vi "StarWarsMelody (SubVI).vi"() -> (3 "Array":dbl[][](array[numeric]))   [LabVIEW 2014]
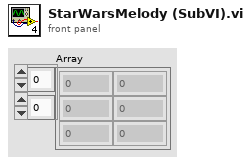
[diagram p1: front panel]
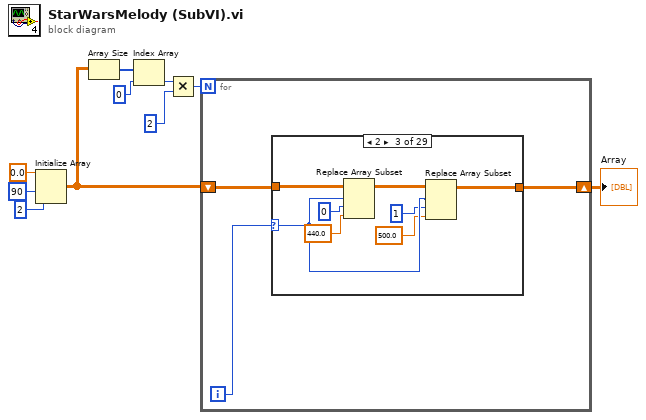
[diagram p0: block diagram]
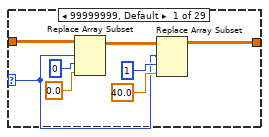
[diagram p2: hidden frame]
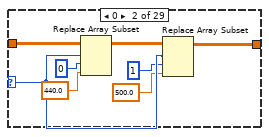
[diagram p3: hidden frame]
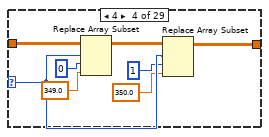
[diagram p4: hidden frame]
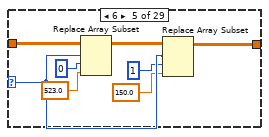
[diagram p5: hidden frame]
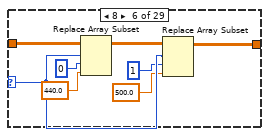
[diagram p6: hidden frame]
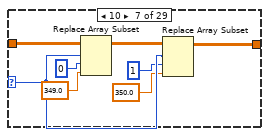
[diagram p7: hidden frame]
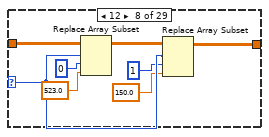
[diagram p8: hidden frame]
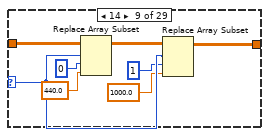
[diagram p9: hidden frame]
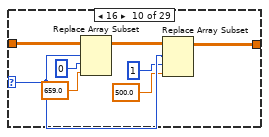
[diagram p10: hidden frame]
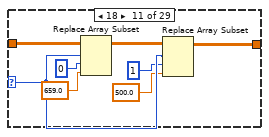
[diagram p11: hidden frame]
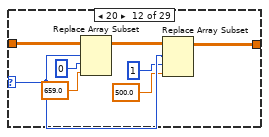
[diagram p12: hidden frame]
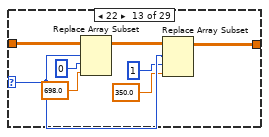
[diagram p13: hidden frame]
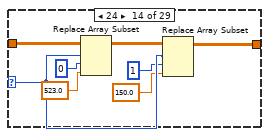
[diagram p14: hidden frame]
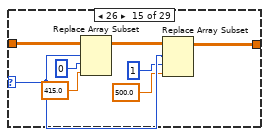
[diagram p15: hidden frame]
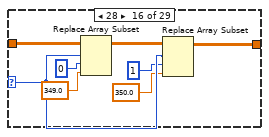
[diagram p16: hidden frame]
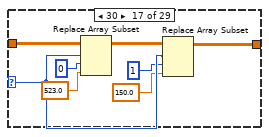
[diagram p17: hidden frame]
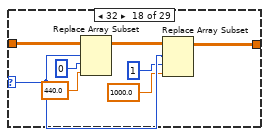
[diagram p18: hidden frame]
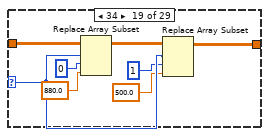
[diagram p19: hidden frame]
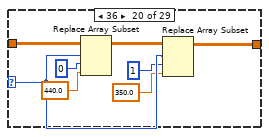
[diagram p20: hidden frame]
diagram:
  n1 = Initialize Array(0.0 ("element"), 90 ("dimension size"), 2 ("dimension size")) -> (w8:dbl[][])
  n2 = Array Size(array=w8) -> (size(s)=w9:i32[])
  n3 = Index Array(array=w9, index=0) -> (element=w3:i32)
  n4 = Multiply(x=w3, y=2) -> (x*y=w4:i32)
  n5 = for {
    N: w4 -> [_]
    shift-right: [w12] -> w1
    shift-left: w8 -> [w13]
    i -> [w11]
    n6 = case shown="2" w11 {
      selector: w11 -> [w14 w25 w33 w41 w49 w57 w65 w73 w81 w89 w97 w105 w113 w121 w129 w137 w145 w153 w161 w169 w177 w185 w193 w201 w209 w217 w225 w233 w241]
      tunnel: w13 -> [w15 w29 w37 w45 w53 w61 w69 w77 w85 w93 w101 w109 w117 w125 w133 w141 w149 w157 w165 w173 w181 w189 w197 w205 w213 w221 w229 w237 w245]
      tunnel: [w16 w22 w30 w38 w46 w54 w62 w70 w78 w86 w94 w102 w110 w118 w126 w134 w142 w150 w158 w166 w174 w182 w190 w198 w206 w214 w222 w230 w238] -> w12
      frame 99999999, Default {
        n7 = Replace Array Subset(array=w15, new element=0.0 ("new element/subarray"), index (row)=w14, index (col)=0 ("disabled index (col)")) -> (w19:dbl[][])
        n8 = Replace Array Subset(array=w19, new element=40.0 ("new element/subarray"), index (row)=w14, index (col)=1 ("disabled index (col)")) -> (w16:dbl[][])
      }
      frame 0 {
        n9 = Replace Array Subset(array=w29, new element=440.0 ("new element/subarray"), index (row)=w25, index (col)=0 ("disabled index (col)")) -> (w26:dbl[][])
        n10 = Replace Array Subset(array=w26, new element=500.0 ("new element/subarray"), index (row)=w25, index (col)=1 ("disabled index (col)")) -> (w22:dbl[][])
      }
      frame 2 {
        n11 = Replace Array Subset(array=w37, new element=440.0 ("new element/subarray"), index (row)=w33, index (col)=0 ("disabled index (col)")) -> (w34:dbl[][])
        n12 = Replace Array Subset(array=w34, new element=500.0 ("new element/subarray"), index (row)=w33, index (col)=1 ("disabled index (col)")) -> (w30:dbl[][])
      }
      frame 4 {
        n13 = Replace Array Subset(array=w45, new element=349.0 ("new element/subarray"), index (row)=w41, index (col)=0 ("disabled index (col)")) -> (w42:dbl[][])
        n14 = Replace Array Subset(array=w42, new element=350.0 ("new element/subarray"), index (row)=w41, index (col)=1 ("disabled index (col)")) -> (w38:dbl[][])
      }
      frame 6 {
        n15 = Replace Array Subset(array=w53, new element=523.0 ("new element/subarray"), index (row)=w49, index (col)=0 ("disabled index (col)")) -> (w50:dbl[][])
        n16 = Replace Array Subset(array=w50, new element=150.0 ("new element/subarray"), index (row)=w49, index (col)=1 ("disabled index (col)")) -> (w46:dbl[][])
      }
      frame 8 {
        n17 = Replace Array Subset(array=w61, new element=440.0 ("new element/subarray"), index (row)=w57, index (col)=0 ("disabled index (col)")) -> (w58:dbl[][])
        n18 = Replace Array Subset(array=w58, new element=500.0 ("new element/subarray"), index (row)=w57, index (col)=1 ("disabled index (col)")) -> (w54:dbl[][])
      }
      frame 10 {
        n19 = Replace Array Subset(array=w69, new element=349.0 ("new element/subarray"), index (row)=w65, index (col)=0 ("disabled index (col)")) -> (w66:dbl[][])
        n20 = Replace Array Subset(array=w66, new element=350.0 ("new element/subarray"), index (row)=w65, index (col)=1 ("disabled index (col)")) -> (w62:dbl[][])
      }
      frame 12 {
        n21 = Replace Array Subset(array=w77, new element=523.0 ("new element/subarray"), index (row)=w73, index (col)=0 ("disabled index (col)")) -> (w74:dbl[][])
        n22 = Replace Array Subset(array=w74, new element=150.0 ("new element/subarray"), index (row)=w73, index (col)=1 ("disabled index (col)")) -> (w70:dbl[][])
      }
      frame 14 {
        n23 = Replace Array Subset(array=w85, new element=440.0 ("new element/subarray"), index (row)=w81, index (col)=0 ("disabled index (col)")) -> (w82:dbl[][])
        n24 = Replace Array Subset(array=w82, new element=1000.0 ("new element/subarray"), index (row)=w81, index (col)=1 ("disabled index (col)")) -> (w78:dbl[][])
      }
      frame 16 {
        n25 = Replace Array Subset(array=w93, new element=659.0 ("new element/subarray"), index (row)=w89, index (col)=0 ("disabled index (col)")) -> (w90:dbl[][])
        n26 = Replace Array Subset(array=w90, new element=500.0 ("new element/subarray"), index (row)=w89, index (col)=1 ("disabled index (col)")) -> (w86:dbl[][])
      }
      frame 18 {
        n27 = Replace Array Subset(array=w101, new element=659.0 ("new element/subarray"), index (row)=w97, index (col)=0 ("disabled index (col)")) -> (w98:dbl[][])
        n28 = Replace Array Subset(array=w98, new element=500.0 ("new element/subarray"), index (row)=w97, index (col)=1 ("disabled index (col)")) -> (w94:dbl[][])
      }
      frame 20 {
        n29 = Replace Array Subset(array=w109, new element=659.0 ("new element/subarray"), index (row)=w105, index (col)=0 ("disabled index (col)")) -> (w106:dbl[][])
        n30 = Replace Array Subset(array=w106, new element=500.0 ("new element/subarray"), index (row)=w105, index (col)=1 ("disabled index (col)")) -> (w102:dbl[][])
      }
      frame 22 {
        n31 = Replace Array Subset(array=w117, new element=698.0 ("new element/subarray"), index (row)=w113, index (col)=0 ("disabled index (col)")) -> (w114:dbl[][])
        n32 = Replace Array Subset(array=w114, new element=350.0 ("new element/subarray"), index (row)=w113, index (col)=1 ("disabled index (col)")) -> (w110:dbl[][])
      }
      frame 24 {
        n33 = Replace Array Subset(array=w125, new element=523.0 ("new element/subarray"), index (row)=w121, index (col)=0 ("disabled index (col)")) -> (w122:dbl[][])
        n34 = Replace Array Subset(array=w122, new element=150.0 ("new element/subarray"), index (row)=w121, index (col)=1 ("disabled index (col)")) -> (w118:dbl[][])
      }
      frame 26 {
        n35 = Replace Array Subset(array=w133, new element=415.0 ("new element/subarray"), index (row)=w129, index (col)=0 ("disabled index (col)")) -> (w130:dbl[][])
        n36 = Replace Array Subset(array=w130, new element=500.0 ("new element/subarray"), index (row)=w129, index (col)=1 ("disabled index (col)")) -> (w126:dbl[][])
      }
      frame 28 {
        n37 = Replace Array Subset(array=w141, new element=349.0 ("new element/subarray"), index (row)=w137, index (col)=0 ("disabled index (col)")) -> (w138:dbl[][])
        n38 = Replace Array Subset(array=w138, new element=350.0 ("new element/subarray"), index (row)=w137, index (col)=1 ("disabled index (col)")) -> (w134:dbl[][])
      }
      frame 30 {
        n39 = Replace Array Subset(array=w149, new element=523.0 ("new element/subarray"), index (row)=w145, index (col)=0 ("disabled index (col)")) -> (w146:dbl[][])
        n40 = Replace Array Subset(array=w146, new element=150.0 ("new element/subarray"), index (row)=w145, index (col)=1 ("disabled index (col)")) -> (w142:dbl[][])
      }
      frame 32 {
        n41 = Replace Array Subset(array=w157, new element=440.0 ("new element/subarray"), index (row)=w153, index (col)=0 ("disabled index (col)")) -> (w154:dbl[][])
        n42 = Replace Array Subset(array=w154, new element=1000.0 ("new element/subarray"), index (row)=w153, index (col)=1 ("disabled index (col)")) -> (w150:dbl[][])
      }
      frame 34 {
        n43 = Replace Array Subset(array=w165, new element=880.0 ("new element/subarray"), index (row)=w161, index (col)=0 ("disabled index (col)")) -> (w162:dbl[][])
        n44 = Replace Array Subset(array=w162, new element=500.0 ("new element/subarray"), index (row)=w161, index (col)=1 ("disabled index (col)")) -> (w158:dbl[][])
      }
      frame 36 {
        n45 = Replace Array Subset(array=w173, new element=440.0 ("new element/subarray"), index (row)=w169, index (col)=0 ("disabled index (col)")) -> (w170:dbl[][])
        n46 = Replace Array Subset(array=w170, new element=350.0 ("new element/subarray"), index (row)=w169, index (col)=1 ("disabled index (col)")) -> (w166:dbl[][])
      }
      frame 38 {
        n47 = Replace Array Subset(array=w181, new element=440.0 ("new element/subarray"), index (row)=w177, index (col)=0 ("disabled index (col)")) -> (w178:dbl[][])
        n48 = Replace Array Subset(array=w178, new element=150.0 ("new element/subarray"), index (row)=w177, index (col)=1 ("disabled index (col)")) -> (w174:dbl[][])
      }
      frame 40 {
        n49 = Replace Array Subset(array=w189, new element=880.0 ("new element/subarray"), index (row)=w185, index (col)=0 ("disabled index (col)")) -> (w186:dbl[][])
        n50 = Replace Array Subset(array=w186, new element=550.0 ("new element/subarray"), index (row)=w185, index (col)=1 ("disabled index (col)")) -> (w182:dbl[][])
      }
      frame 42 {
        n51 = Replace Array Subset(array=w197, new element=830.0 ("new element/subarray"), index (row)=w193, index (col)=0 ("disabled index (col)")) -> (w194:dbl[][])
        n52 = Replace Array Subset(array=w194, new element=250.0 ("new element/subarray"), index (row)=w193, index (col)=1 ("disabled index (col)")) -> (w190:dbl[][])
      }
      frame 44 {
        n53 = Replace Array Subset(array=w205, new element=784.0 ("new element/subarray"), index (row)=w201, index (col)=0 ("disabled index (col)")) -> (w202:dbl[][])
        n54 = Replace Array Subset(array=w202, new element=250.0 ("new element/subarray"), index (row)=w201, index (col)=1 ("disabled index (col)")) -> (w198:dbl[][])
      }
      frame 46 {
        n55 = Replace Array Subset(array=w213, new element=740.0 ("new element/subarray"), index (row)=w209, index (col)=0 ("disabled index (col)")) -> (w210:dbl[][])
        n56 = Replace Array Subset(array=w210, new element=125.0 ("new element/subarray"), index (row)=w209, index (col)=1 ("disabled index (col)")) -> (w206:dbl[][])
      }
      frame 48 {
        n57 = Replace Array Subset(array=w221, new element=698.0 ("new element/subarray"), index (row)=w217, index (col)=0 ("disabled index (col)")) -> (w218:dbl[][])
        n58 = Replace Array Subset(array=w218, new element=125.0 ("new element/subarray"), index (row)=w217, index (col)=1 ("disabled index (col)")) -> (w214:dbl[][])
      }
      frame 50 {
        n59 = Replace Array Subset(array=w229, new element=740.0 ("new element/subarray"), index (row)=w225, index (col)=0 ("disabled index (col)")) -> (w226:dbl[][])
        n60 = Replace Array Subset(array=w226, new element=250.0 ("new element/subarray"), index (row)=w225, index (col)=1 ("disabled index (col)")) -> (w222:dbl[][])
      }
      frame 52 {
        n61 = Replace Array Subset(array=w237, new element=0.0 ("new element/subarray"), index (row)=w233, index (col)=0 ("disabled index (col)")) -> (w234:dbl[][])
        n62 = Replace Array Subset(array=w234, new element=250.0 ("new element/subarray"), index (row)=w233, index (col)=1 ("disabled index (col)")) -> (w230:dbl[][])
      }
      frame 54 {
        n63 = Replace Array Subset(array=w245, new element=0.0 ("new element/subarray"), index (row)=w241, index (col)=0 ("disabled index (col)")) -> (w242:dbl[][])
        n64 = Replace Array Subset(array=w242, new element=0.0 ("new element/subarray"), index (row)=w241, index (col)=1 ("disabled index (col)")) -> (w238:dbl[][])
      }
    }
  }
  "Array" <- w1
